vi "Get XY from Waveform.vi"(1 "Waveform In":waveform(dbl)) -> (0 "XY Array Out":cluster{"Yo":dbl, "Xo":timestamp}[](array[cluster]))   [LabVIEW 2014]
uses:
  <vilib>/Waveform/WDTOps.llb/WDT Get Waveform Time Array DBL.vi
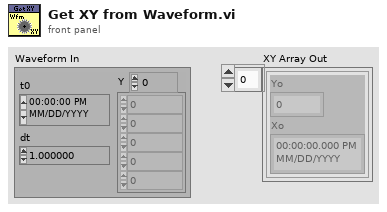
[diagram p1: front panel]
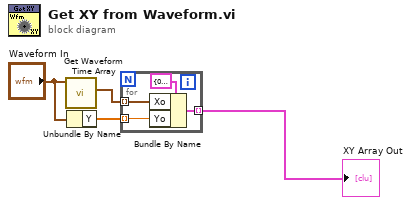
[diagram p0: block diagram]
diagram:
  n1 = call-poly <vilib>:"Get Waveform Time Array.vi"("waveform in"="Waveform In") -> ("X array"=w2:timestamp[])  [unwired: 9 in, 1 out]
  n2 = Unbundle By Name("Waveform In") -> ("Y"=w1:dbl[])
  n3 = for {
    tunnel: w2 -> [w8] mode=indexing
    tunnel: w1 -> [w7] mode=indexing
    tunnel: [w6] -> w4 mode=indexing
    n4 = Bundle By Name(cluster=cluster{"Yo":dbl, "Xo":timestamp} {"Yo"=0.0, "Xo"=timestamp(0 s since 1904-01-01)} ("input cluster"), "Xo"=w8, "Yo"=w7) -> (w6:cluster{"Yo":dbl, "Xo":timestamp})
  }
  "XY Array Out" <- w4
